vi "adjust_filename.vi"(2 "error in":errorcluster, 3 "typeIN":string, 4 "FilePath IN":path) -> (0 "error out":errorcluster, 1 "FilePath OUT":path)   [LabVIEW 2020]
uses:
  <userlib>/_OpenG.lib/file/file.llb/File Exists - Scalar__ogtk.vi
panel:
  out "name":string
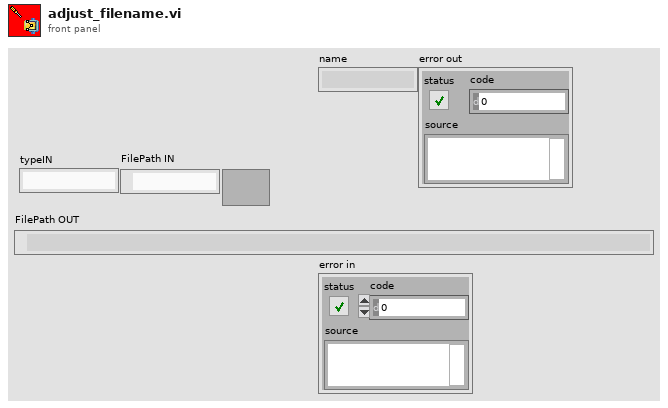
[diagram p1: front panel]
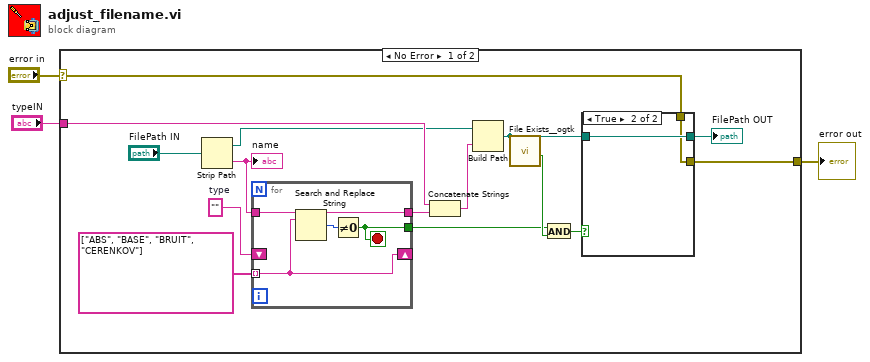
[diagram p0: block diagram]
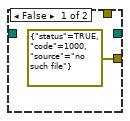
[diagram p2: hidden frame]
diagram:
  n1 = case shown="No Error" "error in" {
    selector: "error in" -> [w4 w27]
    tunnel: "typeIN" -> [w14 _]
    tunnel: [w6 w27] -> w2
    frame No Error {
      w15 = ""  # type
      n2 = Strip Path(path="FilePath IN") -> (stripped path=w11:path, name=w16:string)
      "name" <- w16
      n3 = for {
        tunnel: string[] ["ABS", "BASE", "BRUIT", "CERENKOV"] ("Array") -> [w24] mode=indexing
        tunnel: w16 -> [w26]
        shift-right: [w24] -> _
        shift-left: w15 -> [_]
        tunnel: [w23] -> w13
        tunnel: [w22] -> w5
        stop <- w22 stop-if-true
        n4 = Search and Replace String(input string=w26, search string=w24) -> (result string=w23:string, number of replacements=w25:i32)  [unwired: 6 in, 2 out]
        n5 = Not Equal To 0?(x=w25) -> (x != 0?=w22:bool)
      }
      n6 = Concatenate Strings(w14, w13) -> (w12:string)
      n7 = Build Path(base path=w11, name or relative path=w12) -> (appended path=w9:path)
      n8 = call-poly <userlib>:"File Exists__ogtk.vi"("file path"=w9) -> ("exists"=w8:bool)  [unwired: 6 in, 1 out]
      n9 = And(x=w5, y=w8) -> (x .and. y?=w7:bool)
      n10 = case shown="True" w7 {
        tunnel: [_ w21] -> w10
        tunnel: w9 -> [_ w21]
        tunnel: [errorcluster {"status"=TRUE, "code"=1000, "source"="no such file"} ("error in (no error)") w20] -> w6
        tunnel: w4 -> [_ w20]
        frame False {
        }
        frame True {
        }
      }
      "FilePath OUT" <- w10
    }
    frame Error {
    }
  }
  "error out" <- w2
